vi "kloehn_get_sample.vi"(1 "sample volume":i32 min=0 step=100, 2 "Sample Port":u16(ring) items=["A"=1, "B"=2, "C"=3, "D"=4, "E"=5, "F"=6, "G"=7, "H"=8], 3 "kloehn session in":T1={"VISA resource out"="COM12", "error out"={"status"=FALSE, "code"=0, "source"=""}}) -> (0 "kloehn session out":T1={"VISA resource out"="COM12", "error out"={"status"=FALSE, "code"=0, "source"=""}})   [LabVIEW 2010]
panel:
  # "The VI leaves the syringe on valve on A so that when it is time to inject that can happen immediately and pass on control to the rest of the program flow."
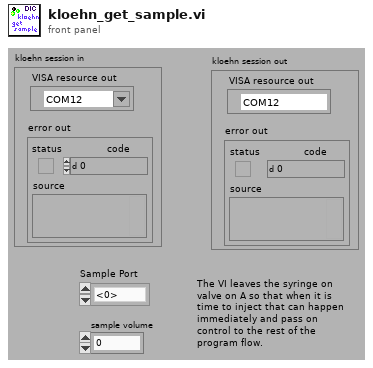
[diagram p1: front panel]
types:
  T1 = cluster{"VISA resource out":refnum<visa-resource-name>, "error out":errorcluster}
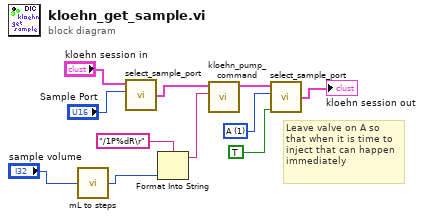
[diagram p0: block diagram]
diagram:
  w4 = u16 1 items=["A"=1, "B"=2, "C"=3, "D"=4, "E"=5, "F"=6, "G"=7, "H"=8] ("Sample Port 2")
  # "Leave valve on A so that when it is time to inject that can happen immediately"
  n1 = call "mL to steps.vi"("mL in"="sample volume") -> ("steps out"=w1:i32)
  n2 = call "select_sample_port.vi"("Sample Port"="Sample Port", "kloehn session in"="kloehn session in") -> ("kloehn session out"=w10:T1)  [unwired: 2 in]
  n3 = Format Into String(format string="/1P%dR\r", w1) -> (resulting string=w7:string)  [unwired: 2 in, 1 out]
  n4 = call "kloehn_pump_command.vi"("Send String"=w7, "kloehn session in"=w10) -> ("kloehn session out"=w6:T1)  [unwired: 6 in, 3 out]
  n5 = call "select_sample_port.vi"("counter-clockwise?"=TRUE, "Sample Port"=w4, "kloehn session in"=w6) -> ("kloehn session out"=→"kloehn session out":T1)  [unwired: 1 in]
